vi "moveComplete-M2.vi"(4 "User Parameter":variant, 5 "Event Data":cluster{"lChanID":i32}, 6 "Control Ref":refnum<k7>, 7 "Event Common Data":T1) -> ()   [LabVIEW 2021]
doc: "André Romero - 2023\nandretec@ifsc.usp.br\nIFSC - USP"
uses:
  Global Motors.vi
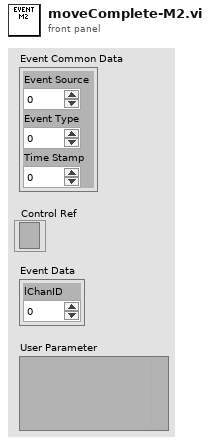
[diagram p1: front panel]
types:
  T1 = cluster{"Event Source":i32, "Event Type":u32, "Time Stamp":u32}
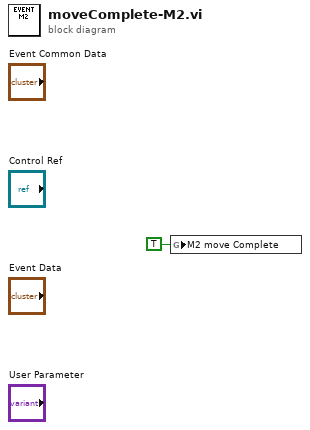
[diagram p0: block diagram]
diagram:
  n1 = global write "Global Motors.vi" "M2 move Complete"(TRUE ("M2 move Complete")) -> ()
